vi "Write Busy.vi"(8 "error in (no error)":errorcluster, 10 "Busy":bool, 11 "Process State Data in":refnum<class "Process State Data.lvclass">) -> (0 "error out":errorcluster, 3 "Process State Data out":refnum<class "Process State Data.lvclass">)   [LabVIEW 2022 SP3, in "Process State Data.lvclass"]
uses:
  Process State Data.lvclass
  Process State Data.lvclass/Process State Data.ctl
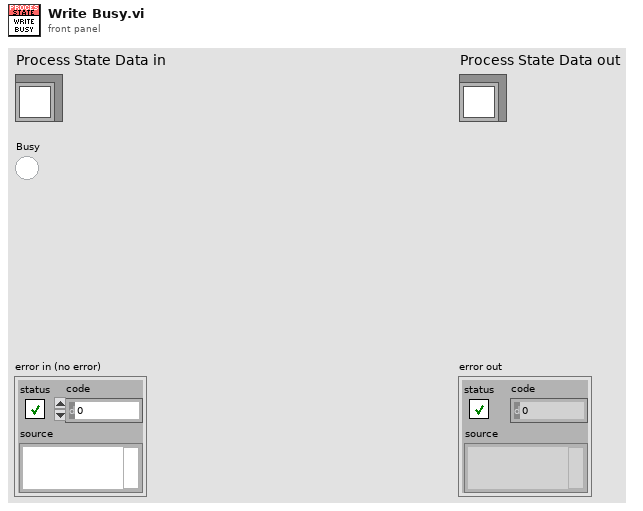
[diagram p1: front panel]
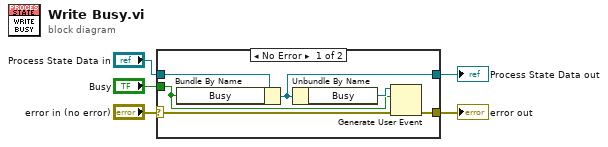
[diagram p0: block diagram]
diagram:
  n1 = case shown="No Error" "error in (no error)" {
    selector: "error in (no error)" -> [w7 w12]
    tunnel: [w6 w12] -> w4
    tunnel: [w10 w13] -> w2
    tunnel: "Process State Data in" -> [w11 w13]
    tunnel: "Busy" -> [w8 _]
    frame No Error {
      n2 = Bundle By Name(cluster=w11, "Busy"=w8) -> (w10:refnum<class "Process State Data.lvclass">)
      n3 = Unbundle By Name(w10) -> ("Busy"=w9:refnum<user-event>)
      n4 = Generate User Event(user event=w9, event data cluster=w8, error in=w7) -> (error out=w6:errorcluster)  [unwired: 1 in, 1 out]
    }
    frame Error {
    }
  }
  "error out" <- w4
  "Process State Data out" <- w2
